vi "test PID with wrappers.vi"() -> ()   [LabVIEW 2011]
panel:
  in  "setpoint 2":dbl=80.0
  in  "stop":bool
  in  "setpoint":dbl=50.0
  out "Waveform Chart":cluster{dbl, dbl}(graph)
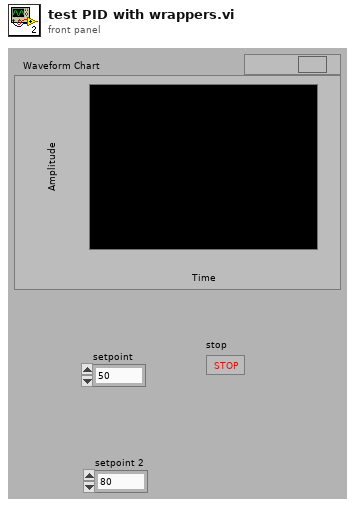
[diagram p1: front panel]
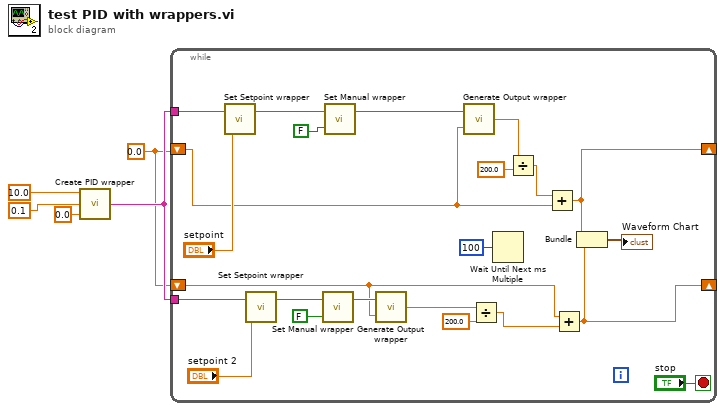
[diagram p0: block diagram]
diagram:
  w1 = 0.0
  n1 = call "Create PID wrapper.vi"("D"=0.0, "I"=0.1, "P"=10.0) -> ("PIDClass string"=w2:string)
  n2 = while {
    tunnel: w2 -> [w17]
    shift-right: [w19] -> _
    shift-left: w1 -> [w10]
    tunnel: w2 -> [w14]
    shift-right: [w20] -> _
    shift-left: w1 -> [w7]
    stop <- "stop" stop-if-true
    n3 = call "Set Setpoint wrapper.vi"("setpoint"="setpoint", "PIDClass string"=w17) -> ("PIDClass string out"=w16:string)
    n4 = call "Set Setpoint wrapper.vi"("setpoint"="setpoint 2", "PIDClass string"=w14) -> ("PIDClass string out"=w11:string)
    n5 = call "Set Manual wrapper.vi"("Manual"=FALSE, "PIDClass string"=w11) -> ("PIDClass string out"=w8:string)
    n6 = call "Set Manual wrapper.vi"("Manual"=FALSE, "PIDClass string"=w16) -> ("PIDClass string out"=w9:string)
    n7 = call "Generate Output wrapper.vi"("PIDClass string"=w8, "Input"=w7) -> ("Output"=w6:dbl)  [unwired: 2 out]
    n8 = call "Generate Output wrapper.vi"("PIDClass string"=w9, "Input"=w10) -> ("Output"=w28:dbl)  [unwired: 2 out]
    n9 = Divide(x=w6, y=200.0) -> (x/y=w21:dbl)
    n10 = Wait Until Next ms Multiple(millisecond multiple=u32 100) -> ()  [unwired: 1 out]
    n11 = Divide(x=w28, y=200.0) -> (x/y=w27:dbl)
    n12 = Add(x=w27, y=w10) -> (x+y=w19:dbl)
    n13 = Add(x=w7, y=w21) -> (x+y=w20:dbl)
    n14 = Bundle(w19, w20) -> (→"Waveform Chart":cluster{dbl, dbl})  [unwired: 1 out]
  }
